vi "Module Not Stopped--error.vi"() -> (0 "error out":errorcluster)   [LabVIEW 2020, in "Interfase.lvlib"]
doc: "Outputs an error cluster containing a custom error code indicating the module was unable to synchronize the module finishing its clean up on exit.\n_____\nBased on Delacor QMH Project Template 5.0.0.82."
uses:
  Interfase.lvlib
  <vilib>/Utility/error.llb/Error Cluster From Error Code.vi
  <vilib>/ErrorRing/Error Ring.xnode
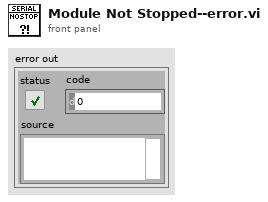
[diagram p1: front panel]
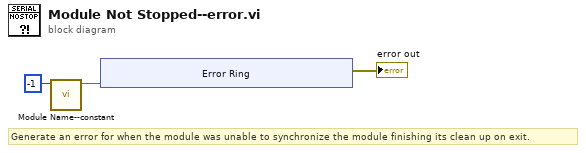
[diagram p0: block diagram]
diagram:
  # "Generate an error for when the module was unable to synchronize the module finishing its clean up on exit."
  n1 = call "Module Name--constant.vi"("Module ID"=-1) -> ("Module Name"=w2:string)  [unwired: 10 in]
  n2 = xnode "Error Ring"("parameter 0"=w2) -> ("error out"=→"error out":errorcluster)
